vi "controlRtOutSignalMode.vi"(7 "Set":bool, 8 "error in":errorcluster, 9 "RT out Mode":enum16{"LVTTL", "LVDS"}(ring), 11 "connection ID":i32) -> (0 "error out":errorcluster, 1 "RT out Mode out":enum16{"LVTTL", "LVDS"}(ring), 3 "connection ID":i32)   [LabVIEW 2016]
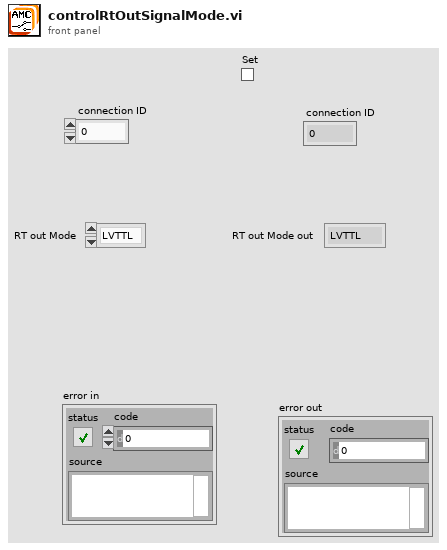
[diagram p1: front panel]
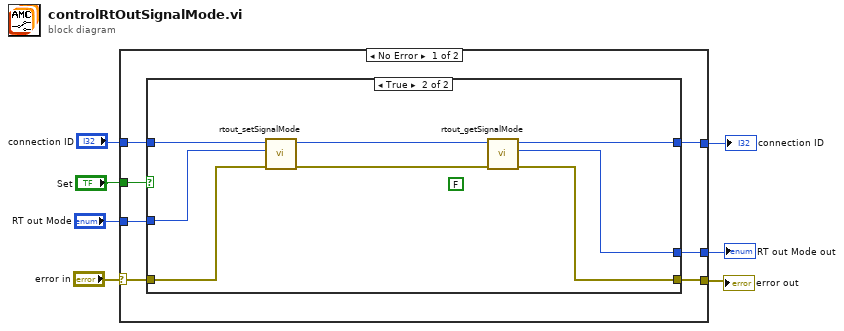
[diagram p0: block diagram]
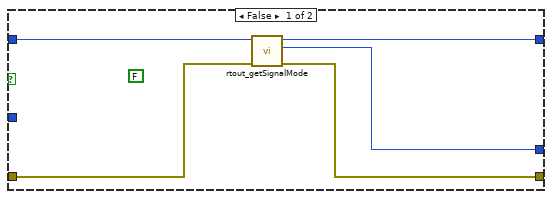
[diagram p2: hidden frame]
diagram:
  n1 = case shown="No Error" "error in" {
    selector: "error in" -> [w8 w29]
    tunnel: [w9 w29] -> w7
    tunnel: "Set" -> [w13 _]
    tunnel: [w11 w28] -> w5
    tunnel: "connection ID" -> [w12 w28]
    tunnel: "RT out Mode" -> [w14 w30]
    tunnel: [w10 w30] -> w2
    frame No Error {
      n2 = case shown="True" w13 {
        tunnel: [w18 w21] -> w11
        tunnel: w12 -> [w19 w27]
        tunnel: [w16 w23] -> w9
        tunnel: [w15 w22] -> w10
        tunnel: w14 -> [_ w25]
        tunnel: w8 -> [w17 w26]
        frame False {
          (unwired) FALSE ("tempvalue")
          n3 = call "rtout_getSignalMode.vi"("error in"=w17, "connection ID"=w19) -> ("error out"=w16:errorcluster, "mode"=w15:i32, "connection ID"=w18:i32)  [unwired: 7 in]
        }
        frame True {
          (unwired) FALSE ("tempvalue")
          n4 = call "rtout_setSignalMode.vi"("error in"=w26, "mode"=w25, "connection ID"=w27) -> ("error out"=w24:errorcluster, "connection ID"=w20:i32)  [unwired: 7 in]
          n5 = call "rtout_getSignalMode.vi"("error in"=w24, "connection ID"=w20) -> ("error out"=w23:errorcluster, "mode"=w22:i32, "connection ID"=w21:i32)  [unwired: 7 in]
        }
      }
    }
    frame Error {
    }
  }
  "error out" <- w7
  "connection ID" <- w5
  "RT out Mode out" <- w2
